vi "Get Library.vi"(8 "error in":errorcluster, 10 "library name":string, 11 "project refnum in":refnum<vi>) -> (0 "error out":errorcluster, 1 "library found?":bool, 2 "library refnum":refnum<vi>, 3 "project refnum out":refnum<vi>)   [LabVIEW 2021, in "InstrumentStudio Plug-In Editor.lvlib"]
uses:
  InstrumentStudio Plug-In Editor.lvlib
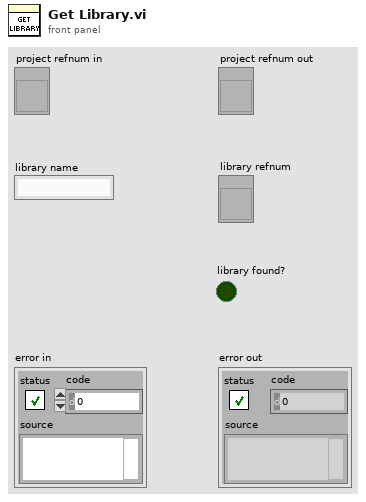
[diagram p1: front panel]
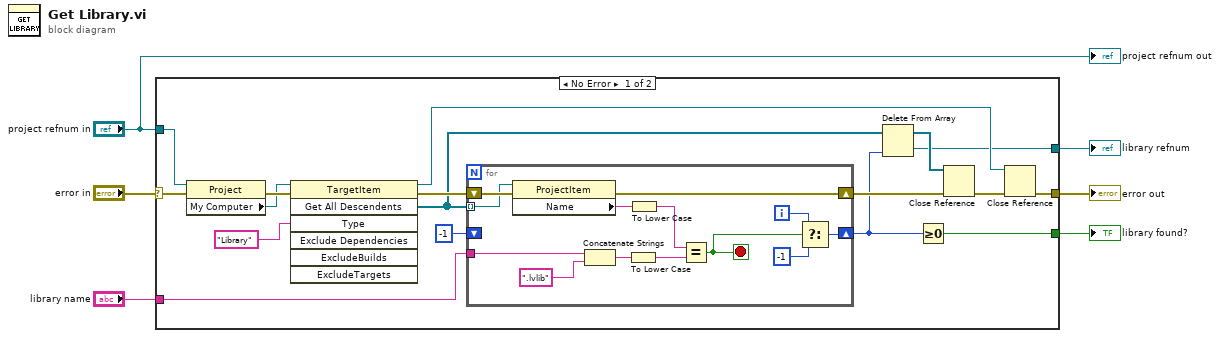
[diagram p0: block diagram]
diagram:
  n1 = case shown="No Error" "error in" {
    selector: "error in" -> [w22 w37]
    tunnel: "project refnum in" -> [w19 _]
    tunnel: [w12 w37] -> w4
    tunnel: [w10 _] -> w3
    tunnel: [w7 _] -> w1
    tunnel: "library name" -> [w13 _]
    frame No Error {
      n2 = property class="Project"(reference=w19, error in=w22) -> (error out=w23:errorcluster, "My Computer"=w18:refnum<vi>)  [unwired: 1 out]
      n3 = invoke class="TargetItem" method="Get All Descendents"(reference=w18, error in=w23, "Type"="Library") -> (reference out=w11:refnum<vi>, error out=w20:errorcluster, "All Descendents"=w16:refnum<vi>[])  [unwired: 4 in, 4 out]
      n4 = for {
        tunnel: w16 -> [w35] mode=indexing
        shift-right: [w30] -> w21
        shift-left: w20 -> [w36]
        tunnel: w13 -> [w34]
        shift-right: [w26] -> w9
        shift-left: -1 ("f") -> [_]
        i -> [w28]
        stop <- w24 stop-if-true
        n5 = property class="ProjectItem"(reference=w35, error in=w36) -> (error out=w30:errorcluster, "Name"=w31:string)  [unwired: 1 out]
        n6 = Concatenate Strings(w34, ".lvlib" ("string")) -> (w32:string)
        n7 = To Lower Case(string=w32) -> (all lower case string=w27:string)
        n8 = To Lower Case(string=w31) -> (all lower case string=w25:string)
        n9 = Equal?(x=w25, y=w27) -> (x = y?=w24:bool)
        n10 = Select(t=w28, s=w24, f=-1) -> (s? t:f=w26:i32)
      }
      n11 = Delete From Array(array=w16, index=w9) -> (deleted portion=w10:refnum<vi>, array with subset deleted=w14:refnum<vi>[])  [unwired: 1 in]
      n12 = Greater Or Equal To 0?(x=w9) -> (x >= 0?=w7:bool)
      n13 = Close Reference(reference=w14, error in (no error)=w21) -> (error out=w15:errorcluster)
      n14 = Close Reference(reference=w11, error in (no error)=w15) -> (error out=w12:errorcluster)
    }
    frame Error {
    }
  }
  "error out" <- w4
  "library refnum" <- w3
  "library found?" <- w1
  "project refnum out" <- "project refnum in"
